vi "Parse ifconfig data.vi"(10 "NIC Name":string, 11 "ifconfig":string="\neth0      Link encap:Ethernet  HWaddr b8:27:eb:a0:af:7b  \n          inet addr:10.2.229.47  Bcast:10.2.229.255  Mask:255.255.255.0\n          inet6 addr: fe80::94d4:326d:3c15:d2d5/64 Scope:Link\n          UP BROADCAST RUNNING MULTICAST  MTU:1500  Metric:1\n          RX packets:408214 errors:0 dropped:1 overruns:0 frame:0\n          TX packets:6889 errors:0 dropped:0 overruns:0 carrier:0\n          collisions:0 txqueuelen:1000 \n          RX bytes:28941251 (27.6 MiB)  TX bytes:966268 (943.6 KiB)\n\nlo        Link encap:Local Loopback  \n          inet addr:127.0.0.1  Mask:255.0.0.0\n          inet6 addr: ::1/128 Scope:Host\n          UP LOOPBACK RUNNING  MTU:65536  Metric:1\n          RX packets:8 errors:0 dropped:0 overruns:0 frame:0\n          TX packets:8 errors:0 dropped:0 overruns:0 carrier:0\n          collisions:0 txqueuelen:0 \n          RX bytes:1104 (1.0 KiB)  TX bytes:1104 (1.0 KiB)\n\nwlan0     Link encap:Ethernet  HWaddr 00:0f:60:07:c0:e5  \n          inet addr:192.168.1.5  Bcast:255.255.255.255  Mask:255.255.255.0\n          inet6 addr: fe80::6361:2767:fd85:6cf1/64 Scope:Link\n          UP BROADCAST RUNNING MULTICAST  MTU:1500  Metric:1\n          RX packets:20125 errors:0 dropped:1 overruns:0 frame:0\n          TX packets:5648 errors:0 dropped:0 overruns:0 carrier:0\n          collisions:0 txqueuelen:1000 \n          RX bytes:5538493 (5.2 MiB)  TX bytes:637437 (622.4 KiB)\n\n") -> (2 "Subnet mask":string, 3 "IP Address":string)   [LabVIEW 2011, in "LMH-LINX.lvlib"]
uses:
  <vilib>/regexp/Match Regular Expression.xnode
  LMH-LINX.lvlib
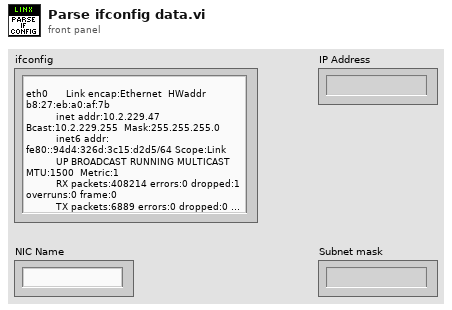
[diagram p1: front panel]
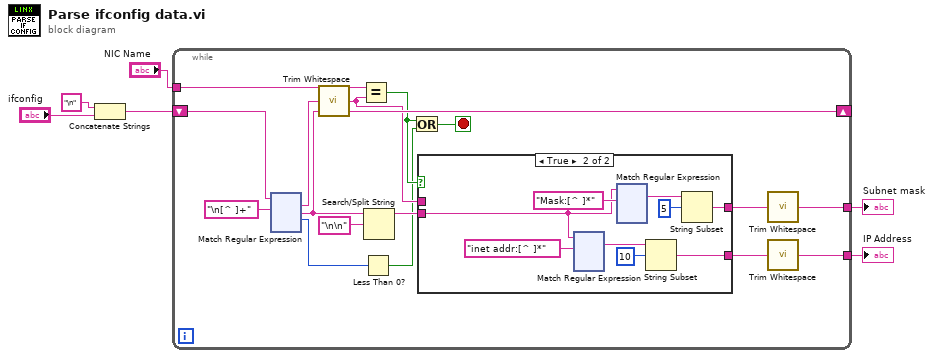
[diagram p0: block diagram]
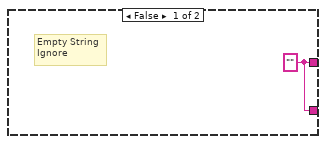
[diagram p2: hidden frame]
diagram:
  n1 = Concatenate Strings("\n" ("string"), "ifconfig") -> (w1:string)
  n2 = while {
    shift-right: [w17] -> _
    shift-left: w1 -> [w22]
    tunnel: "NIC Name" -> [w15]
    tunnel: [w7] -> w4
    tunnel: [w9] -> w5
    stop <- w13 stop-if-true
    n3 = xnode "Match Regular Expression"("input string"=w22, "regular expression"="\n[^ ]+") -> ("whole match"=w14:string, "after match"=w17:string, "offset past match"=w20:i32)  [unwired: 4 in, 2 out]
    n4 = call <vilib>:"Trim Whitespace.vi"("string"=w14) -> ("trimmed string"=w16:string)  [unwired: 1 in]
    n5 = Equal?(x=w15, y=w16) -> (x = y?=w12:bool)
    n6 = Less Than 0?(x=w20) -> (x < 0?=w11:bool)
    n7 = Search/Split String(string=w17, search string/char (-)="\n\n") -> (substring before match=w18:string)  [unwired: 1 in, 2 out]
    n8 = Or(x=w12, y=w11) -> (x .or. y?=w13:bool)
    n9 = case shown="True" w12 {
      tunnel: w16 -> [_ _]
      tunnel: w18 -> [_ w26]
      tunnel: [w23 w25] -> w8
      tunnel: [w23 w24] -> w10
      frame False {
        w23 = "" ("whole match")
        # "Empty String\nIgnore"
      }
      frame True {
        n10 = xnode "Match Regular Expression"("input string"=w26, "regular expression"="inet addr:[^ ]*") -> ("whole match"=w31:string)  [unwired: 4 in, 4 out]
        n11 = xnode "Match Regular Expression"("input string"=w26, "regular expression"="Mask:[^ ]*") -> ("whole match"=w28:string)  [unwired: 4 in, 4 out]
        n12 = String Subset(string=w31, offset (0)=10) -> (substring=w24:string)  [unwired: 1 in]
        n13 = String Subset(string=w28, offset (0)=5) -> (substring=w25:string)  [unwired: 1 in]
      }
    }
    n14 = call <vilib>:"Trim Whitespace.vi"("string"=w8) -> ("trimmed string"=w7:string)  [unwired: 1 in]
    n15 = call <vilib>:"Trim Whitespace.vi"("string"=w10) -> ("trimmed string"=w9:string)  [unwired: 1 in]
  }
  "IP Address" <- w5
  "Subnet mask" <- w4
